vi "18-Explode.vi"(11 "Snailfish Number in":string) -> (2 "Exploded?":bool, 3 "Snailfish Number out":string)   [LabVIEW 2019, in "18.lvlib"]
uses:
  18.lvlib
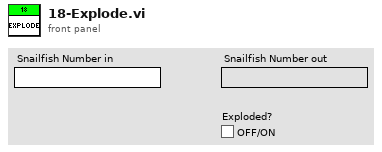
[diagram p1: front panel]
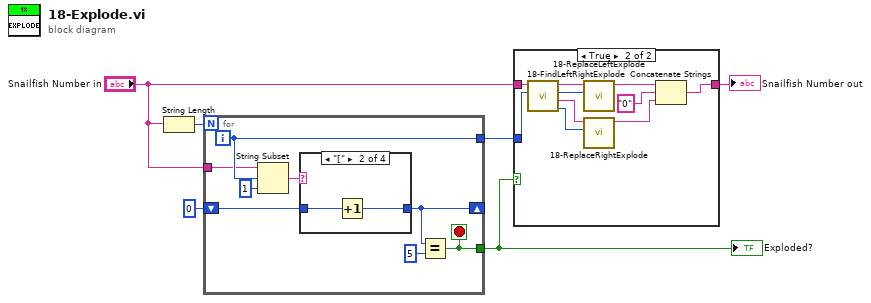
[diagram p0: block diagram]
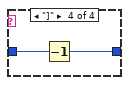
[diagram p5: hidden frame]
diagram:
  n1 = String Length(string="Snailfish Number in") -> (length=w5:i32)
  n2 = for {
    N: w5 -> [_]
    tunnel: "Snailfish Number in" -> [w7]
    shift-right: [w11] -> _
    shift-left: u8 0 ("[") -> [w12]
    tunnel: [w9] -> w4
    tunnel: [w8] -> w1
    i -> [w9]
    stop <- w8 stop-if-true
    n3 = String Subset(string=w7, offset (0)=w9, length (rest)=1 ("length (rest)")) -> (substring=w13:string)
    n4 = case shown="\"[\"" w13 {
      tunnel: w12 -> [w15 w17 w18 w20]
      tunnel: [w15 w16 w18 w19] -> w11
      frame Default {
      }
      frame "[" {
        n5 = Increment(x=w17) -> (x+1=w16:u8)
      }
      frame "," {
      }
      frame "]" {
        n6 = Decrement(x=w20) -> (x-1=w19:u8)
      }
    }
    n7 = Equal?(x=w11, y=u8 5) -> (x = y?=w8:bool)
  }
  "Exploded?" <- w1
  n8 = case shown="True" w1 {
    tunnel: w4 -> [_ w24]
    tunnel: "Snailfish Number in" -> [w21 w23]
    tunnel: [w21 w22] -> w2
    frame False {
    }
    frame True {
      n9 = call "18-FindLeftRightExplode.vi"("Explode Position"=w24, "Snailfish Number in in"=w23) -> ("Right Explosion"=w27:u64, "Right Snailfish Number out"=w25:string, "Left Explosion"=w28:u64, "Left Snailfish Number out"=w29:string)  [unwired: 6 in]
      n10 = call "18-ReplaceLeftExplode.vi"("Left Explosion"=w28, "Left Snailfish Number in"=w29) -> ("Left Snailfish Number out"=w30:string)  [unwired: 9 in]
      n11 = call "18-ReplaceRightExplode.vi"("Right Explosion"=w27, "Right Snailfish Number in"=w25) -> ("Right Snailfish Number out"=w26:string)  [unwired: 9 in]
      n12 = Concatenate Strings(w30, "0" ("string"), w26) -> (w22:string)
    }
  }
  "Snailfish Number out" <- w2
